vi "RespTracker.vi"(4 "Gate Length":i32=250, 6 "Gate Start":i32=-150, 7 "threshold y":dbl=25.0, 8 "AS Med Fil":i32=100, 9 "RF pts to use":i32=1000, 10 "initial Skip index":i32=50, 11 "2-D data array":i16[][](array[numeric])) -> (0 "Resp Gate":bool[](array[boolean]), 1 "RF Threshold":dbl[](graph), 2 "Locations":dbl[](array[numeric]), 3 "All curves":dbl[][](graph))   [LabVIEW 2022 SP3]
uses:
  <vilib>/Analysis/baseanly.llb/Scale 1D.vi
  <vilib>/Analysis/baseanly.llb/Mean (DBL).vi
  <vilib>/Analysis/2dsp.llb/1D Cross Correlation (DBL).vi
  <vilib>/Analysis/NI_AALPro.lvlib
  <vilib>/Analysis/NI_AALBase.lvlib
  <vilib>/Analysis/NI_AAL_SigProc.lvlib
panel:
  out "Raw data":i16[][](graph)
  out "RF Threshold 3":dbl[](graph)
  out "RF Threshold 2":dbl[](graph)
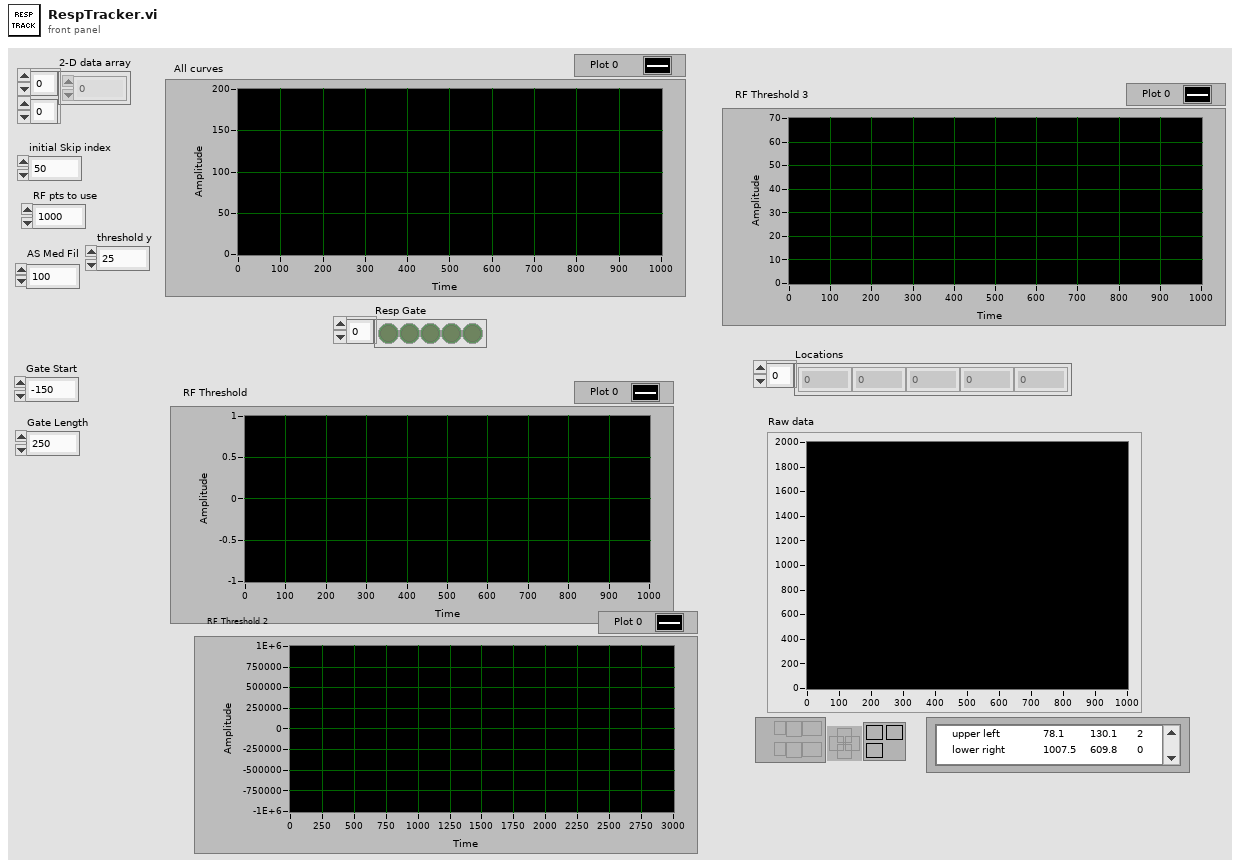
[diagram p1: front panel]
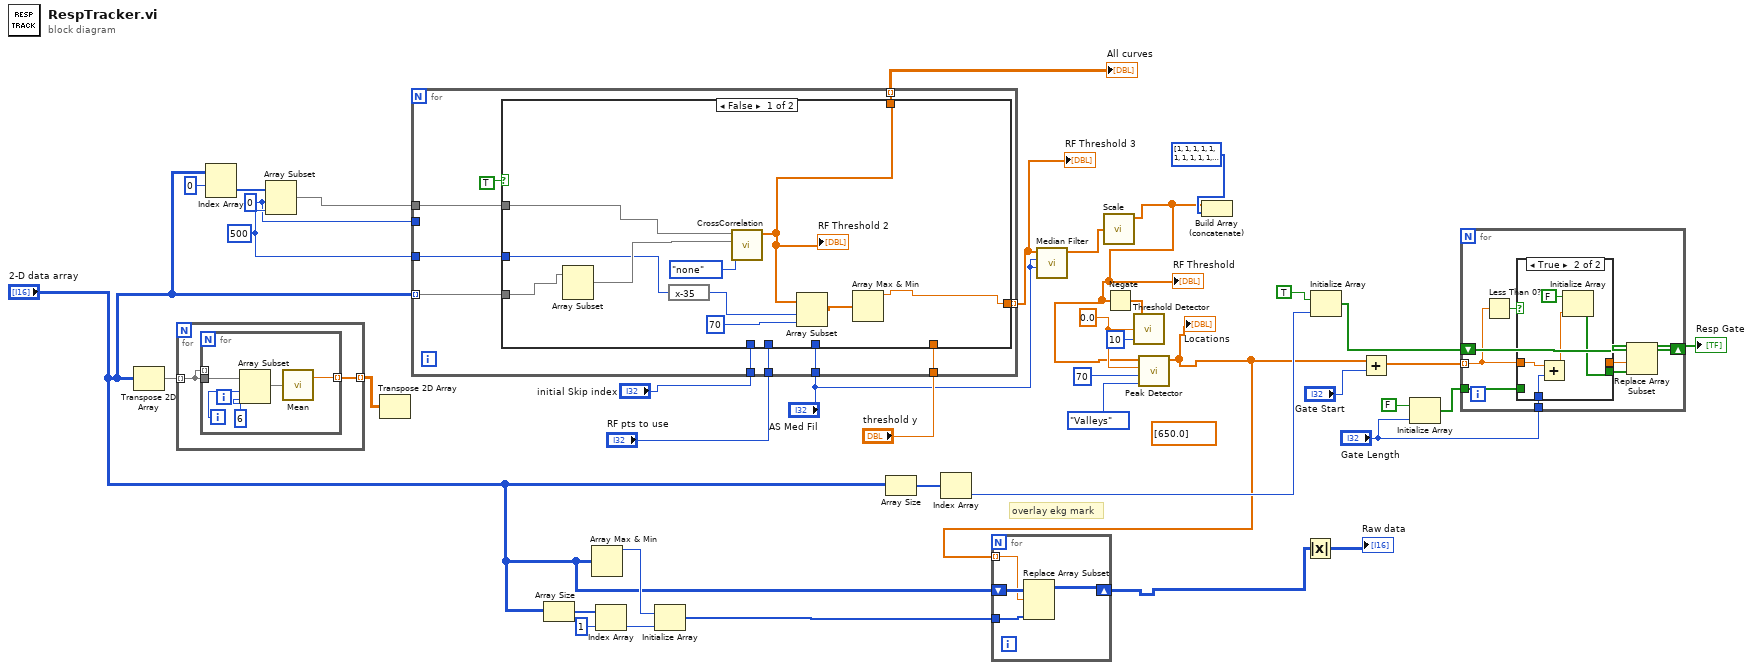
[diagram p0: block diagram]
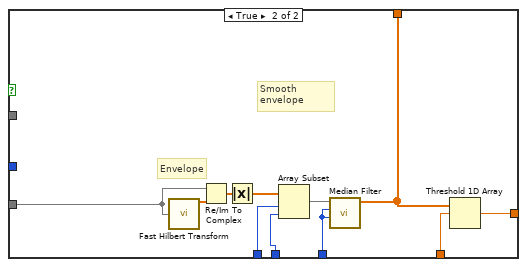
[diagram p3: hidden frame]
diagram:
  w22 = 0 ("index")
  w18 = sgl 0.0 ("width")
  (unwired) dbl[] [650.0] ("Locations")
  w25 = 500 ("length")
  # "overlay ekg mark"
  n1 = Transpose 2D Array(2D array="2-D data array") -> (transposed array=w9:i16[][])
  n2 = for {
    tunnel: w9 -> [w42] mode=indexing
    tunnel: [w41] -> w8 mode=indexing
    n3 = for {
      tunnel: w42 -> [w47]
      tunnel: w42 -> [_] mode=indexing
      tunnel: [w45] -> w41 mode=indexing
      i -> [w44]
      n4 = Array Subset(array=w47, index=w44, length=6) -> (w46:i16[])
      n5 = call-poly <vilib>:"Mean.vi"("X"=w46) -> ("mean"=w45:dbl)  [unwired: 1 out]
    }
  }
  n6 = Index Array(array="2-D data array", index (row)=0) -> (element=w26:i16[])  [unwired: 1 in]
  n7 = Array Subset(array=w26, index=w22, length=w25) -> (w21:i16[])
  n8 = Transpose 2D Array(2D array=w8) -> ()  [unwired: 1 out]
  n9 = for {
    tunnel: "2-D data array" -> [w57] mode=indexing
    tunnel: "RF pts to use" -> [w56]
    tunnel: [w55] -> w6 mode=indexing
    tunnel: [w54] -> w40 mode=indexing
    tunnel: "initial Skip index" -> [w53]
    tunnel: "AS Med Fil" -> [w52]
    tunnel: "threshold y" -> [w51]
    tunnel: w25 -> [w49]
    tunnel: w22 -> [_]
    tunnel: w21 -> [w48]
    n10 = case shown="False" TRUE {
      tunnel: w57 -> [w63 w75]
      tunnel: w56 -> [_ w74]
      tunnel: [w60 w69] -> w55
      tunnel: [w59 w68] -> w54
      tunnel: w53 -> [_ w73]
      tunnel: w52 -> [_ w72]
      tunnel: w51 -> [_ w71]
      tunnel: w49 -> [w61 _]
      tunnel: w48 -> [w64 _]
      frame False {
        n11 = Array Subset(array=w63) -> (w62:i16[])  [unwired: 2 in]
        n12 = expression code="x-35"(w61) -> (w67:i32)
        n13 = call-poly <vilib>:"CrossCorrelation.vi"("normalization"=enum32{"none", "unbiased", "biased"}."none", "Y"=w62, "X"=w64) -> ("Rxy"=w59:dbl[])  [unwired: 7 in, 1 out]
        "RF Threshold 2" <- w59
        n14 = Array Subset(array=w59, index=w67, length=70) -> (w58:dbl[])
        n15 = Array Max & Min(array=w58) -> (max value=w60:dbl)  [unwired: 3 out]
      }
      frame True {
        # "Smooth envelope"
        # "Envelope"
        n16 = call <vilib>:"Fast Hilbert Transform.vi"("X"=w75) -> ("Hilbert{X}"=w77:dbl[])  [unwired: 1 out]
        n17 = Re/Im To Complex(1:w77, 2:w75) -> (0:w76:cdb[])
        n18 = Absolute Value(x=w76) -> (abs(x)=w78:dbl[])
        n19 = Array Subset(array=w78, index=w73, length=w74) -> (w70:dbl[])
        n20 = call <vilib>:"Median Filter.vi"("right rank"=w72, "left rank"=w72, "X"=w70) -> ("Filtered X"=w68:dbl[])  [unwired: 8 out]
        n21 = Threshold 1D Array(2:w71, 3:w68) -> (0:w69:dbl)  [unwired: 1 in]
      }
    }
  }
  "All curves" <- w40
  "RF Threshold 3" <- w6
  n22 = Array Size(array="2-D data array") -> (size(s)=w15:i32[])
  n23 = Array Max & Min(array="2-D data array") -> (max value=w13:i16)  [unwired: 3 out]
  n24 = Index Array(array=w15, index=1) -> (element=w14:i32)
  n25 = Initialize Array(w13, w14) -> (w12:i16[])
  n26 = Array Size(array="2-D data array") -> (size(s)=w32:i32[])
  n27 = Index Array(array=w32) -> (element=w31:i32)  [unwired: 1 in]
  n28 = call <vilib>:"Median Filter.vi"("right rank"="AS Med Fil", "left rank"="AS Med Fil", "X"=w6) -> ("Filtered X"=w5:dbl[])  [unwired: 8 out]
  n29 = call-poly <vilib>:"Scale.vi"("X"=w5) -> ("Y=(X-offset)/scale"=w3:dbl[])  [unwired: 3 out]
  "RF Threshold" <- w3
  n30 = Negate(x=w3) -> (-x=w7:dbl[])
  n31 = call <vilib>:"Threshold Detector.vi"("width"=10, "threshold"=w18, "X"=w7) -> ()  [unwired: 3 out]
  n32 = call <vilib>:"Peak Detector.vi"("peaks/valleys"=enum32{"Peaks", "Valleys"}."Valleys", "width"=70, "threshold"=w18, "X"=w3) -> ("Locations"=w1:dbl[])  [unwired: 3 in, 4 out]
  "Locations" <- w1
  n33 = for {
    tunnel: w1 -> [w80] mode=indexing
    tunnel: w12 -> [w81]
    shift-right: [w79] -> w11
    shift-left: "2-D data array" -> [w82]
    n34 = Replace Array Subset(array=w82, new element=w81, index (row)=w80) -> (w79:i16[][])  [unwired: 1 in]
  }
  n35 = Build Array (concatenate)(w3, i32[] [1, 1, 1, 1, 1, 1, 1, 1, 1, 1, 1, 1, 1, 1, 1, 1, 1, 1, 1, 1, 1]) -> ()  [unwired: 1 out]
  n36 = Absolute Value(x=w11) -> (abs(x)=→"Raw data":i16[][])
  n37 = Initialize Array(TRUE, w31) -> (w34:bool[])
  n38 = Add(x=w1, y="Gate Start") -> (x+y=w37:dbl[])
  n39 = Initialize Array(FALSE, "Gate Length") -> (w35:bool[])
  n40 = for {
    tunnel: w37 -> [w85] mode=indexing
    shift-right: [w89] -> w33
    shift-left: w34 -> [w90]
    tunnel: w35 -> [w86]
    tunnel: "Gate Length" -> [w84]
    n41 = Less Than 0?(x=w85) -> (x < 0?=w88:bool)
    n42 = case shown="True" w88 {
      tunnel: [w92 w93] -> w87
      tunnel: w86 -> [w92 _]
      tunnel: w85 -> [w91 w97]
      tunnel: w84 -> [_ w96]
      tunnel: [w91 _] -> w83
      frame False {
      }
      frame True {
        n43 = Add(x=w97, y=w96) -> (x+y=w94:dbl)
        n44 = Initialize Array(FALSE, w94) -> (w93:bool[])
      }
    }
    n45 = Replace Array Subset(array=w90, new element=w87, index=w83) -> (w89:bool[])
  }
  "Resp Gate" <- w33
